vi "optionsAcq_channel_cycleCountingWavemeter.vi"(6 "readWrite":enum16{"read", "write"}(ring), 8 "error in (no error)":errorcluster, 9 "waveMeter on":bool, 11 "OSAchannel in":refnum<class "OSAchannel.lvclass">) -> (0 "error out":errorcluster, 1 "waveMeter on read":bool, 2 "FTSLib_status":i32, 3 "OSAchannel out":refnum<class "OSAchannel.lvclass">)   [LabVIEW 2010, in "OSAchannel.lvclass"]
uses:
  OSAchannel.lvclass
  OSAchannel.lvclass/OSAchannel.ctl
  _dll/LVLib/FTSLib.lvlib
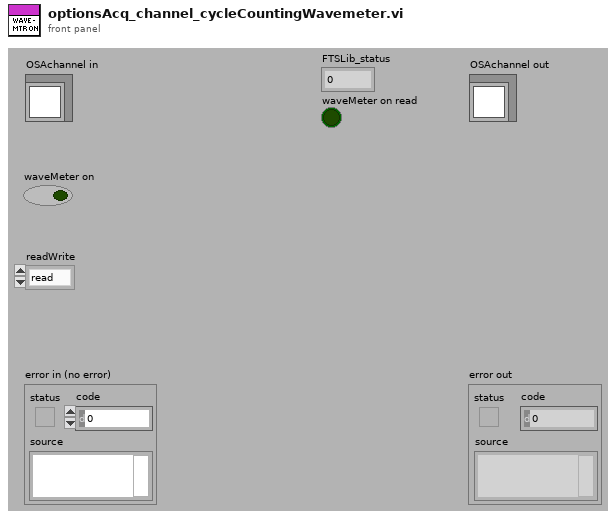
[diagram p1: front panel]
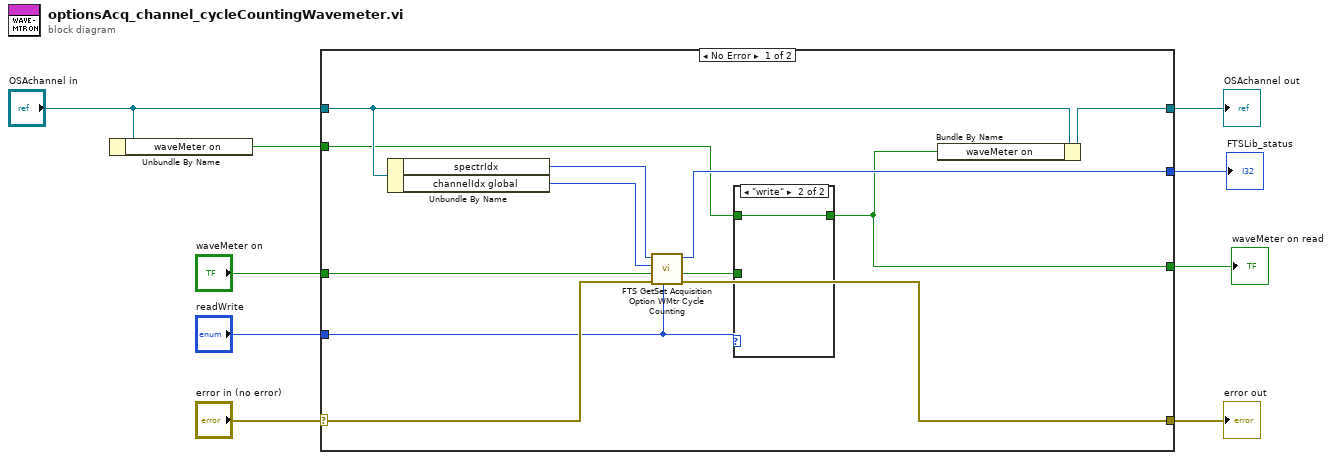
[diagram p0: block diagram]
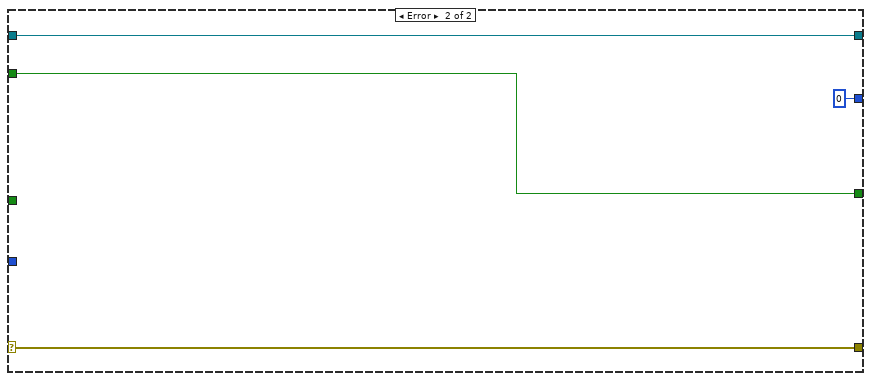
[diagram p3: hidden frame]
diagram:
  n1 = Unbundle By Name("OSAchannel in") -> ("waveMeter on"=w1:bool)
  n2 = case shown="No Error" "error in (no error)" {
    selector: "error in (no error)" -> [w19 w27]
    tunnel: [w18 w27] -> w8
    tunnel: [w14 w26] -> w7
    tunnel: "OSAchannel in" -> [w16 w26]
    tunnel: "waveMeter on" -> [w17 _]
    tunnel: "readWrite" -> [w15 _]
    tunnel: [w12 0 ("FTSLib_status")] -> w4
    tunnel: [w11 w24] -> w3
    tunnel: w1 -> [w10 w24]
    frame No Error {
      n3 = Unbundle By Name(w16) -> ("spectrIdx"=w21:u16, "channelIdx global"=w20:u16)
      n4 = call "FTS GetSet Acquisition Option WMtr Cycle Counting.vi"("readWrite"=w15, "error in"=w19, "cycleCounting"=w17, "channel index interferogram"=w20, "spectrometerIdx"=w21) -> ("error out"=w18:errorcluster, "cycleCounting read"=w13:bool, "FTSLib_status"=w12:i32)  [unwired: 4 in]
      n5 = case shown="\"write\"" w15 {
        tunnel: w10 -> [_ w23]
        tunnel: [w22 w23] -> w11
        tunnel: w13 -> [w22 _]
        frame "read", Default {
        }
        frame "write" {
        }
      }
      n6 = Bundle By Name(cluster=w16, "waveMeter on"=w11) -> (w14:refnum<class "OSAchannel.lvclass">)
    }
    frame Error {
    }
  }
  "error out" <- w8
  "OSAchannel out" <- w7
  "FTSLib_status" <- w4
  "waveMeter on read" <- w3
